vi "ER2007 Data History Panel.vi"() -> ()   [LabVIEW 2013]
uses:
  Controls/Global ER2007.vi
panel:
  in  "T = Update config":bool=TRUE
  in  "Case Constant\n(See Context Help)":bool
  in  "Match Scale":bool
  in  "Cursors 2":bool caption="Cursors"
  in  "AutoScl 2":bool=TRUE caption="AutoScale"
  in  "Cursors 1":bool caption="Cursors"
  in  "AutoScl 1":bool=TRUE caption="Auto Scale"
  in  "Log/Linear":bool
  in  "Print 2":bool
  in  "Print 1":bool
  in  "Export":bool
  out "Cell #":string="<none>"
  out "PV2 Label":string="F 2-3"
  out "Time ER2":dbl format="%.1f"
  out "ER2":dbl format="%.3f"
  out "Time ER1":dbl format="%.1f"
  out "ER1":dbl format="%.3f"
  out "Time PV2":dbl format="%.1f"
  out "Temp/Press":dbl format="%.1f"
  out "Time PV1":dbl format="%.1f"
  out "Pore Volume":dbl format="%.3f"
  out "Table":string[][](table)
  in  "Other PV's":u16(ring)=5 items=["FF 2-3", "Temp A", "Temp B", "Conf P", "Pore P", "Delta-P"]
  in  "ER 2":u16(ring)=2 items=["E-R 1-2", "E-R 1-3", "E-R 1-4", "E-R 2-3"]
  in  "ER 1":u16(ring)=3 items=["E-R 1-2", "E-R 1-3", "E-R 1-4", "E-R 2-3"]
  out "PV XY":cluster{"Y":dbl[], "Y":dbl[]}[](graph)
  in  "Exit":bool
  in  "Graph/Table":bool
  out "Resist XY":cluster{"Y":dbl[], "Y":dbl[]}[](graph)
  # "Data History"
  # "Resistivity Values"
  # "Process Values"
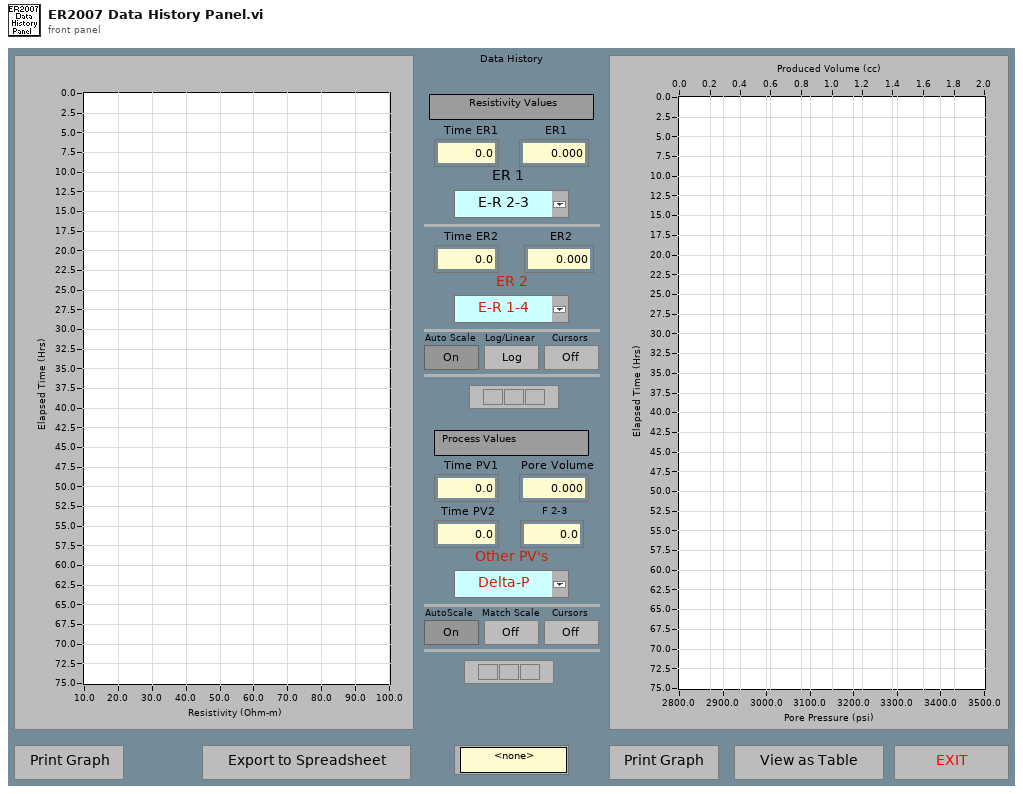
[diagram p1: front panel]
types:
  T1 = enum16{"open", "open or create", "create or replace", "create", "open (read only)"}
  T2 = cluster{"CurCell":i32, "Cell Data":cluster{"Cell ID":i32, "Cell Status":enum16{"Inactive", "Setup", "Active", "Done"}, "Project":string, "Sample #":string, "Rock Type":string, "Fluid Pair":string, "Rw":dbl, "Rw Temp":dbl, "Length":dbl, "Diameter":dbl, "Porosity":dbl, "Permeability":dbl, "4P":bool, "ElectSpace":dbl, "Frequency":dbl, "Amplitude":dbl, "DAQ Period":u32, "DAQ Units":u16, "Start Time":dbl, "Next Time":dbl, "Datafile":path, "Last Pore Vol":dbl, "Last Pore Xdcr":enum16{"<none>", "Lo Range", "Hi Range"}, "Last Resistor":enum16{"<none>", "Resistor 1", "Resistor 2", "Resistor 3", "Resistor 4", "Resistor 5", "Resistor 6"}, "CurData":dbl[][], "Comment":string}[]}
  T3 = cluster{"Cell ID":i32, "Cell Status":enum16{"Inactive", "Setup", "Active", "Done"}, "Project":string, "Sample #":string, "Rock Type":string, "Fluid Pair":string, "Rw":dbl, "Rw Temp":dbl, "Length":dbl, "Diameter":dbl, "Porosity":dbl, "Permeability":dbl, "4P":bool, "ElectSpace":dbl, "Frequency":dbl, "Amplitude":dbl, "DAQ Period":u32, "DAQ Units":u16, "Start Time":dbl, "Next Time":dbl, "Datafile":path, "Last Pore Vol":dbl, "Last Pore Xdcr":enum16{"<none>", "Lo Range", "Hi Range"}, "Last Resistor":enum16{"<none>", "Resistor 1", "Resistor 2", "Resistor 3", "Resistor 4", "Resistor 5", "Resistor 6"}, "CurData":dbl[][], "Comment":string}[]
  T4 = cluster{"Cell ID":i32, "Cell Status":enum16{"Inactive", "Setup", "Active", "Done"}, "Project":string, "Sample #":string, "Rock Type":string, "Fluid Pair":string, "Rw":dbl, "Rw Temp":dbl, "Length":dbl, "Diameter":dbl, "Porosity":dbl, "Permeability":dbl, "4P":bool, "ElectSpace":dbl, "Frequency":dbl, "Amplitude":dbl, "DAQ Period":u32, "DAQ Units":u16, "Start Time":dbl, "Next Time":dbl, "Datafile":path, "Last Pore Vol":dbl, "Last Pore Xdcr":enum16{"<none>", "Lo Range", "Hi Range"}, "Last Resistor":enum16{"<none>", "Resistor 1", "Resistor 2", "Resistor 3", "Resistor 4", "Resistor 5", "Resistor 6"}, "CurData":dbl[][], "Comment":string}
  T5 = cluster{"ER-1":u16, "ER-2":u16, "PV-Top":u16, "PV-Bot":u16, "GraphCfg":cluster{"AutoScl":bool, "T-Hi":dbl, "T-Lo":dbl, "PV-Hi":dbl, "PV-Lo":dbl}[]}
  T6 = cluster{"AutoScl":bool, "T-Hi":dbl, "T-Lo":dbl, "PV-Hi":dbl, "PV-Lo":dbl}[]
  T7 = cluster{"AutoScl":bool, "T-Hi":dbl, "T-Lo":dbl, "PV-Hi":dbl, "PV-Lo":dbl}
  T8 = typedef "LVPointDoubleTypeDef.ctl" = cluster{"Cursor X":dbl, "Cursor Y":dbl}
  T9 = typedef "LVRangeTypeDef.ctl" = cluster{"Minimum":dbl, "Maximum":dbl, "Increment":dbl, "Minor Increment":dbl, "Start":dbl}
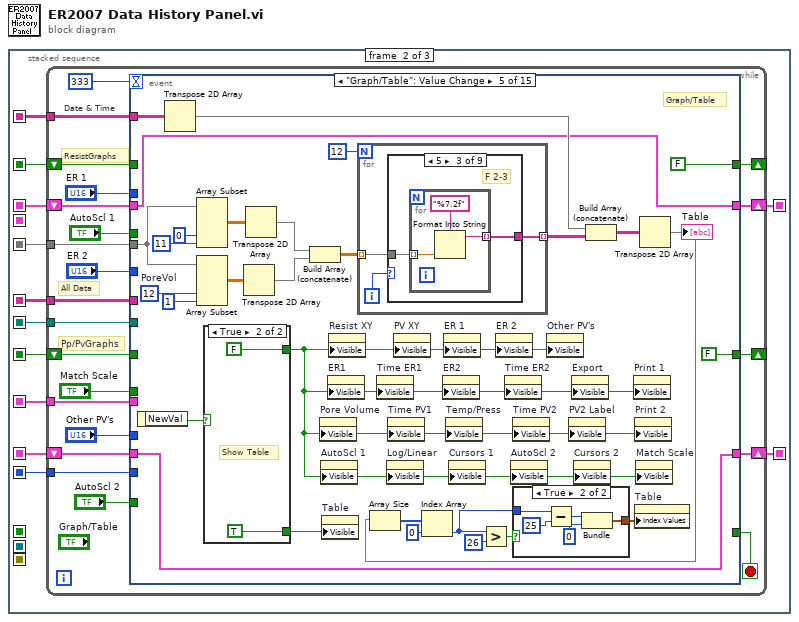
[diagram p0: block diagram]
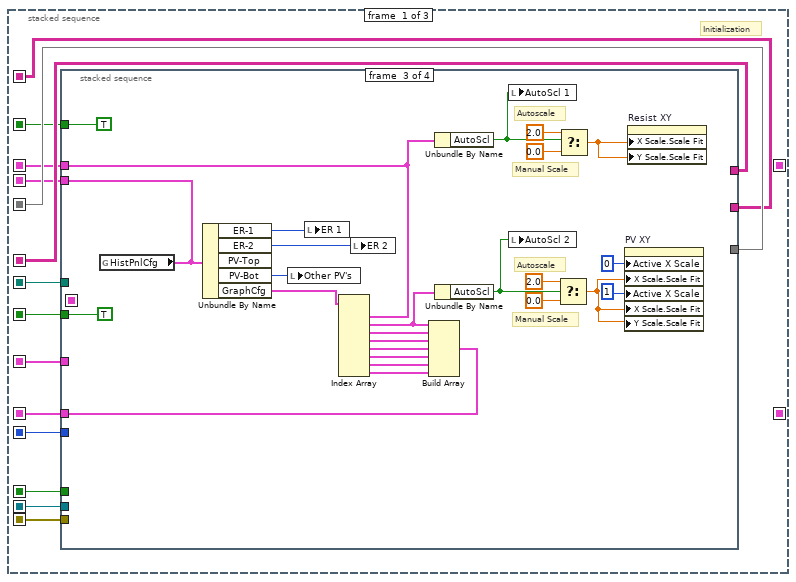
[diagram p2: hidden frame]
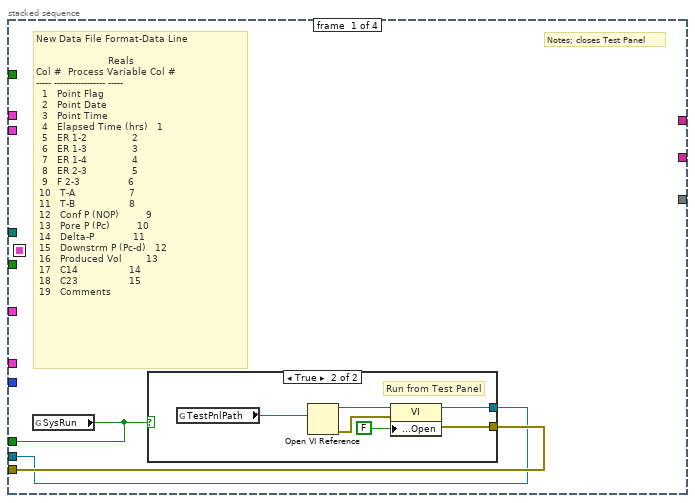
[diagram p3: hidden frame]
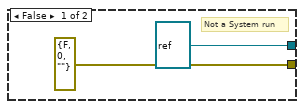
[diagram p4: hidden frame]
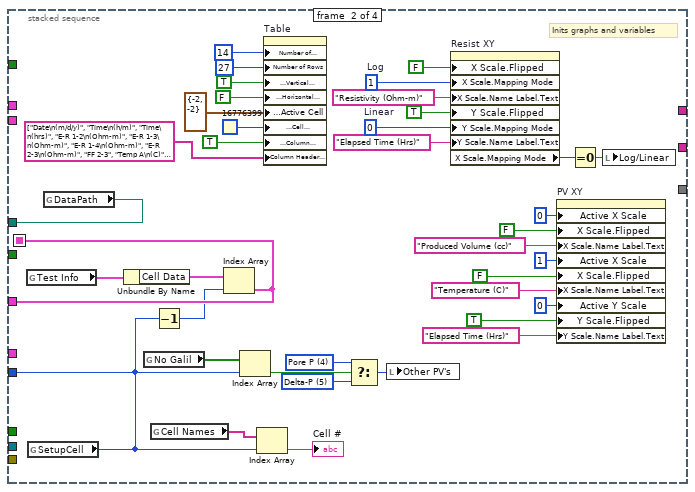
[diagram p5: hidden frame]
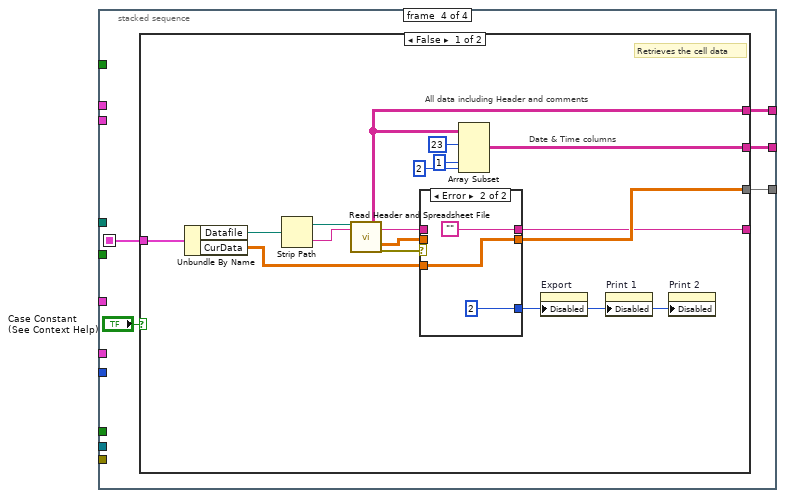
[diagram p6: hidden frame]
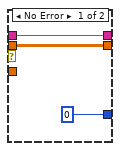
[diagram p7: hidden frame]
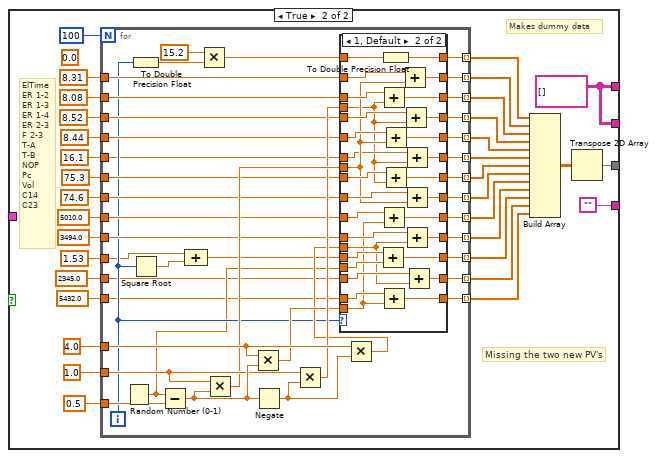
[diagram p8: hidden frame]
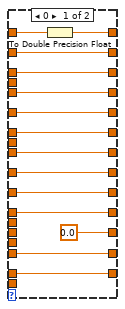
[diagram p9: hidden frame]
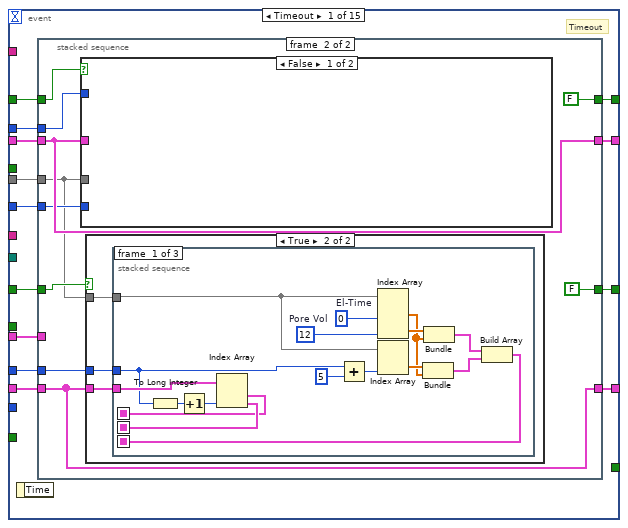
[diagram p10: hidden frame]
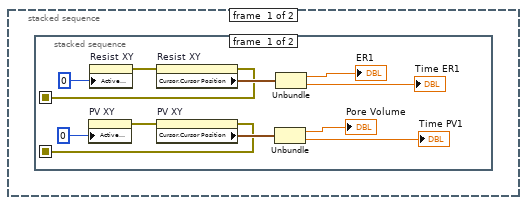
[diagram p11: hidden frame]
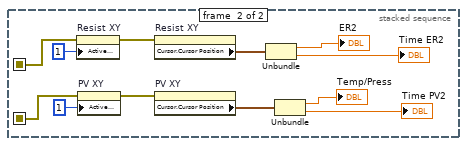
[diagram p12: hidden frame]
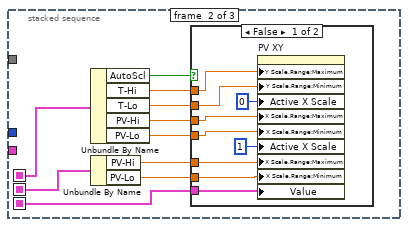
[diagram p14: hidden frame]
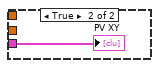
[diagram p15: hidden frame]
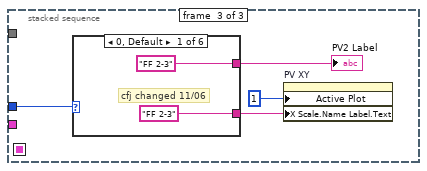
[diagram p16: hidden frame]
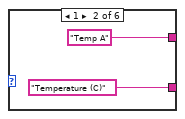
[diagram p17: hidden frame]
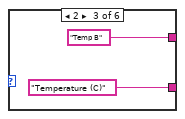
[diagram p18: hidden frame]
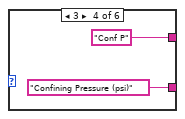
[diagram p19: hidden frame]
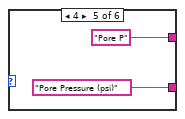
[diagram p20: hidden frame]
diagram:
  n1 = stacked-sequence {
    seq-local: [w10 _ _] -> [_ w247 _]
    seq-local: [w14 _ _] -> [_ _ w844]
    seq-local: [w13 _ _] -> [_ _ w843]
    seq-local: [w12 _ _] -> [_ _ w842]
    seq-local: [w11 _ _] -> [_ w246 _]
    seq-local: [w9 _ _] -> [_ w245 _]
    seq-local: [w8 _ _] -> [_ w244 _]
    seq-local: [w7 _ _] -> [_ w243 _]
    seq-local: [w6 _ _] -> [_ w242 _]
    seq-local: [w5 _ _] -> [_ _ w841]
    seq-local: [w2 _ _] -> [_ w240 _]
    seq-local: [w4 _ _] -> [_ w239 _]
    seq-local: [w3 _ _] -> [_ w241 _]
    seq-local: [w1 _ _] -> [_ w238 _]
    seq-local: [_ w236 _] -> [_ _ w840]
    seq-local: [_ w237 _] -> [_ _ w839]
    frame #0 {
      # "Initialization"
      n2 = stacked-sequence {
        seq-local: [_ w43 _ _] -> [_ _ _ w92]
        tunnel: [_ _ _ w94] -> w10
        tunnel: [w16 _ _ _] -> w14
        tunnel: [w15 _ _ _] -> w13
        tunnel: [w17 _ _ _] -> w12
        tunnel: [_ w43 _ _] -> w11
        tunnel: [_ w30 _ _] -> w9
        tunnel: [_ w40 _ _] -> w8
        tunnel: [_ _ _ w91] -> w7
        tunnel: [_ _ _ w90] -> w6
        tunnel: [_ _ w89 _] -> w5
        tunnel: [_ _ TRUE _] -> w4
        tunnel: [_ _ TRUE _] -> w3
        tunnel: [_ _ w82 _] -> w2
        tunnel: [_ _ w74 _] -> w1
        frame #0 {
          # "New Data File Format-Data Line\n\n                        Reals\nCol #  Process Variable Col #\n----- ----------------- -----\n  1   Point Flag\n  2   Point Date\n  3   Point Time\n  4   Elapsed Time (hrs)   1\n  5   ER 1-2               2\n  6   ER 1-3               3\n  7   ER 1-4               4\n  8   ER 2-3               5\n  9   F 2-3                6\n 10   T-A                  7\n 11   T-B                  8\n 12   Conf P (NOP)         9\n 13   Pore P (Pc)         10\n 14   Delta-P             11\n 15   Downstrm P (Pc-d)   12\n 16   Produced Vol        13\n 17   C14                 14\n 18   C23                 15\n 19   Comments"
          # "Notes; closes Test Panel"
          n3 = global read "Global ER2007.vi" "SysRun"() -> (w16:bool)
          n4 = case shown="True" w16 {
            tunnel: [refnum<vi> refnum w22] -> w15
            tunnel: [errorcluster {"status"=FALSE, "code"=0, "source"=""} ("error out") w21] -> w17
            frame False {
              # "Not a System run"
            }
            frame True {
              # "Run from Test Panel"
              n5 = global read "Global ER2007.vi" "TestPnlPath"() -> (w20:path)
              n6 = Open VI Reference(vi path=w20) -> (vi reference=w25:refnum<vi>, error out=w24:errorcluster)  [unwired: 5 in]
              n7 = property class="VI"(reference=w25, error in=w24, "Front Panel Window:Open"=FALSE) -> (reference out=w22:refnum<vi>, error out=w21:errorcluster)
            }
          }
        }
        frame #1 {
          w28 = u16 4 items=["FF 2-3", "Temp A", "Temp B", "Conf P", "Pore P", "Delta-P"] ("Other PV's")
          w27 = u16 5 items=["FF 2-3", "Temp A", "Temp B", "Conf P", "Pore P", "Delta-P"] ("Other PV's")
          w54 = u8 0  # Linear
          w55 = u8 1  # Log
          # "Inits graphs and variables"
          n8 = global read "Global ER2007.vi" "Test Info"() -> (w39:T2)
          n9 = global read "Global ER2007.vi" "SetupCell"() -> (w30:i32)
          n10 = global read "Global ER2007.vi" "DataPath"() -> (w40:path)
          n11 = Unbundle By Name(w39) -> ("Cell Data"=w44:T3)
          n12 = global read "Global ER2007.vi" "No Galil"() -> (w31:bool[])
          n13 = global read "Global ER2007.vi" "Cell Names"() -> (w38:string[])
          n14 = Decrement(x=w30) -> (x-1=w36:i32)
          n15 = Index Array(array=w44, index=w36) -> (element=w43:T4)
          n16 = Index Array(array=w31, index=w30) -> (element=w29:bool)
          n17 = Index Array(array=w38, index=w30) -> (element=→"Cell #":string)
          n18 = property on="Table" class="Tbl (strict)"("Number of Columns"=u32 14, "Number of Rows"=u32 27, "Visible Items:Vertical Scrollbar Visible"=TRUE ("Vertical Scrollbar Visible"), "Visible Items:Horizontal Scrollbar Visible"=FALSE ("Horizontal Scrollbar Visible"), "Active Cell:Active Cell"=cluster{"Row":i32, "Column":i32} {"Row"=-2, "Column"=-2} ("Active Cell"), "Active Cell:Cell Background Color"=u32 16776399, "Visible Items:Column Headers Visible"=TRUE ("Column Headers Visible"), "Column Header Strings[]"=string[] ["Date\n(m/d/y)", "Time\n(h/m)", "Time\n(hrs)", "E-R 1-2\n(Ohm-m)", "E-R 1-3\n(Ohm-m)", "E-R 1-4\n(Ohm-m)", "E-R 2-3\n(Ohm-m)", "FF 2-3", "Temp A\n(C)", "Temp B\n(C)", "Conf P\n(psi)", "Pore P\n(psi)", "Delta-P\n(psi)", "Prod Vol\n(cc)"] ("Column Headers[]")) -> ()  [unwired: 2 in, 2 out]
          n19 = Select(t=w28, s=w29, f=w27) -> (s? t:f=w26:u16)
          n20 = local write "Other PV's"(w26) -> ()
          n21 = property on="Resist XY" class="XYGraph (strict)"("X Scale.Flipped"=FALSE, "X Scale.Mapping Mode"=w55, "X Scale.Name Label.Text"="Resistivity (Ohm-m)", "Y Scale.Flipped"=TRUE, "Y Scale.Mapping Mode"=w54, "Y Scale.Name Label.Text"="Elapsed Time (Hrs)") -> ("X Scale.Mapping Mode"=w41:u8)  [unwired: 2 in, 2 out]
          n22 = property on="PV XY" class="XYGraph (strict)"("Active X Scale"=0, "X Scale.Flipped"=FALSE, "X Scale.Name Label.Text"="Produced Volume (cc)", "Active X Scale"=1, "X Scale.Flipped"=FALSE, "X Scale.Name Label.Text"="Temperature (C)", "Active Y Scale"=0, "Y Scale.Flipped"=TRUE, "Y Scale.Name Label.Text"="Elapsed Time (Hrs)") -> ()  [unwired: 2 in, 2 out]
          n23 = Equal To 0?(x=w41) -> (x = 0?=w42:bool)
          n24 = local write "Log/Linear"(w42) -> ()
        }
        frame #2 {
          # "Manual Scale"
          # "Manual Scale"
          # "Autoscale"
          # "Autoscale"
          n25 = global read "Global ER2007.vi" "HistPnlCfg"() -> (w89:T5)
          n26 = Unbundle By Name(w89) -> ("ER-1"=w86:u16, "ER-2"=w85:u16, "PV-Bot"=w84:u16, "GraphCfg"=w83:T6)  [unwired: 1 out]
          n27 = local write "Other PV's"(w84) -> ()
          n28 = local write "ER 1"(w86) -> ()
          n29 = Index Array(array=w83) -> (element #1=w82:T7, element #2=w75:T7, element #3=w81:T7, element #4=w80:T7, element #5=w79:T7, element #6=w78:T7, element #7=w77:T7, element #8=w76:T7)  [unwired: 8 in]
          n30 = local write "ER 2"(w85) -> ()
          n31 = Build Array(w75, w81, w80, w79, w78, w77, w76) -> (w74:T6)
          n32 = Unbundle By Name(w82) -> ("AutoScl"=w69:bool)
          n33 = Unbundle By Name(w75) -> ("AutoScl"=w68:bool)
          n34 = local write "AutoScl 1"(w69) -> ()
          n35 = local write "AutoScl 2"(w68) -> ()
          n36 = Select(t=2.0, s=w68, f=0.0) -> (s? t:f=w64:dbl)
          n37 = Select(t=2.0, s=w69, f=0.0) -> (s? t:f=w67:dbl)
          n38 = property on="PV XY" class="XYGraph (strict)"("Active X Scale"=0, "X Scale.Scale Fit"=w64, "Active X Scale"=1, "X Scale.Scale Fit"=w64, "Y Scale.Scale Fit"=w64) -> ()  [unwired: 2 in, 2 out]
          n39 = property on="Resist XY" class="XYGraph (strict)"("X Scale.Scale Fit"=w67, "Y Scale.Scale Fit"=w67) -> ()  [unwired: 2 in, 2 out]
        }
        frame #3 {
          n40 = case shown="False" "Case Constant\n(See Context Help)" {
            tunnel: [w102 w126] -> w94
            tunnel: w92 -> [w110 _]
            tunnel: [w101 ""] -> _
            tunnel: [w96 w117] -> w91
            tunnel: [w95 w117] -> w90
            frame False {
              # "All data including Header and comments"
              # "Date & Time columns"
              # "Retrieves the cell data"
              n41 = Unbundle By Name(w110) -> ("Datafile"=w109:path, "CurData"=w104:dbl[][])
              n42 = Strip Path(path=w109) -> (stripped path=w108:path, name=w107:string)
              n43 = call "Read Header and Spreadsheet File.vi"("DirIn"=w108, "NameIn"=w107) -> ("Table Out"=w96:string[][], "File Text Out"=w103:string, "2D Data"=w105:sgl[][], "Error Out"=w106:errorcluster)  [unwired: 11 in, 3 out]
              n44 = case shown="Error" w106 {
                tunnel: [w113 w116] -> w102
                tunnel: w105 -> [w113 _]
                tunnel: w104 -> [_ w116]
                tunnel: w103 -> [w112 _]
                tunnel: [w112 ""] -> w101
                tunnel: [u8 0 ("Disabled") u8 2 ("Disabled")] -> w100
                frame No Error {
                }
                frame Error {
                }
              }
              n45 = Array Subset(array=w96, index (row)=23 ("index"), index (col)=1 ("index"), length (col)=2 ("length")) -> (w95:string[][])  [unwired: 1 in]
              n46 = property on="Export" class="Bool"("Disabled"=w100) -> ()  [unwired: 2 in, 2 out]
              n47 = property on="Print 1" class="Bool"("Disabled"=w100) -> ()  [unwired: 2 in, 2 out]
              n48 = property on="Print 2" class="Bool"("Disabled"=w100) -> ()  [unwired: 2 in, 2 out]
            }
            frame True {
              w117 = string[][] [] ("Table Out")
              (unwired) 0.0 ("y")
              # "Missing the two new PV's"
              # "Makes dummy data"
              # "ElTime\nER 1-2\nER 1-3\nER 1-4\nER 2-3\nF 2-3\nT-A\nT-B\nNOP\nPc\nVol\nC14\nC23"
              n49 = for {
                N: 100 -> [_]
                tunnel: 0.5 ("y") -> [w190]
                tunnel: 1.0 ("y") -> [w188]
                tunnel: 4.0 ("y") -> [w187]
                tunnel: [w185] -> w131 mode=indexing
                tunnel: 8.31 ("y") -> [w181]
                tunnel: [w180] -> w130 mode=indexing
                tunnel: 8.08 ("y") -> [w178]
                tunnel: [w177] -> w129 mode=indexing
                tunnel: 8.52 ("y") -> [w175]
                tunnel: [w174] -> w128 mode=indexing
                tunnel: 8.44 ("y") -> [w173]
                tunnel: [w172] -> w137 mode=indexing
                tunnel: 75.3 ("y") -> [w171]
                tunnel: [w170] -> w136 mode=indexing
                tunnel: 74.6 ("y") -> [w169]
                tunnel: [w168] -> w135 mode=indexing
                tunnel: 5010.0 ("y") -> [w167]
                tunnel: [w166] -> w134 mode=indexing
                tunnel: 3494.0 ("y") -> [w165]
                tunnel: [w164] -> w133 mode=indexing
                tunnel: [w163] -> w132 mode=indexing
                tunnel: 1.53 ("value") -> [w156]
                tunnel: 16.1 ("y") -> [w155]
                tunnel: [w154] -> w123 mode=indexing
                tunnel: 2345.0 ("value") -> [w153]
                tunnel: 5432.0 ("value") -> [w152]
                tunnel: [w151] -> w120 mode=indexing
                tunnel: [w150] -> w119 mode=indexing
                i -> [w159]
                n50 = Random Number (0-1)() -> (number: 0 to 1=w157:dbl)
                n51 = To Double Precision Float(number=w159) -> (double precision float=w182:dbl)
                n52 = Square Root(x=w159) -> (sqrt(x)=w158:dbl)
                n53 = Subtract(x=w157, y=w190) -> (x-y=w189:dbl)
                n54 = Compound Arithmetic op=ADD(w156, w158) -> (w160:dbl)
                n55 = Multiply(x=15.2, y=w182) -> (x*y=w184:dbl)
                n56 = Multiply(x=w188, y=w189) -> (x*y=w179:dbl)
                n57 = Multiply(x=w187, y=w189) -> (x*y=w162:dbl)
                n58 = Negate(x=w189) -> (-x=w186:dbl)
                n59 = Multiply(x=w188, y=w186) -> (x*y=w176:dbl)
                n60 = Multiply(x=w187, y=w186) -> (x*y=w161:dbl)
                n61 = case shown="1, Default" w159 {
                  tunnel: w184 -> [w204 w235]
                  tunnel: [w203 w234] -> w185
                  tunnel: w181 -> [w202 w232]
                  tunnel: [w202 w233] -> w180
                  tunnel: w179 -> [_ w221]
                  tunnel: w178 -> [w201 w230]
                  tunnel: [w201 w231] -> w177
                  tunnel: w176 -> [_ w213]
                  tunnel: w175 -> [w200 w228]
                  tunnel: [w200 w229] -> w174
                  tunnel: w173 -> [w199 w226]
                  tunnel: [w199 w227] -> w172
                  tunnel: w171 -> [w198 w224]
                  tunnel: [w198 w225] -> w170
                  tunnel: w169 -> [w197 w222]
                  tunnel: [w197 w223] -> w168
                  tunnel: w167 -> [w196 w219]
                  tunnel: [w196 w220] -> w166
                  tunnel: w165 -> [w195 w217]
                  tunnel: [w195 w218] -> w164
                  tunnel: w160 -> [_ w216]
                  tunnel: [0.0 w211] -> w163
                  tunnel: w162 -> [_ w205]
                  tunnel: w161 -> [_ w206]
                  tunnel: w157 -> [_ w215]
                  tunnel: w155 -> [w191 w214]
                  tunnel: [w191 w212] -> w154
                  tunnel: w153 -> [w193 w210]
                  tunnel: w152 -> [w192 w209]
                  tunnel: [w193 w208] -> w151
                  tunnel: [w192 w207] -> w150
                  frame 0 {
                    n62 = To Double Precision Float(number=w204) -> (double precision float=w203:dbl)
                  }
                  frame 1, Default {
                    n63 = Add(x=w216, y=w215) -> (x+y=w211:dbl)
                    n64 = Add(x=w230, y=w213) -> (x+y=w231:dbl)
                    n65 = Add(x=w219, y=w205) -> (x+y=w220:dbl)
                    n66 = Add(x=w209, y=w205) -> (x+y=w207:dbl)
                    n67 = To Double Precision Float(number=w235) -> (double precision float=w234:dbl)
                    n68 = Add(x=w226, y=w221) -> (x+y=w227:dbl)
                    n69 = Add(x=w224, y=w213) -> (x+y=w225:dbl)
                    n70 = Add(x=w232, y=w221) -> (x+y=w233:dbl)
                    n71 = Add(x=w228, y=w213) -> (x+y=w229:dbl)
                    n72 = Add(x=w214, y=w213) -> (x+y=w212:dbl)
                    n73 = Add(x=w222, y=w221) -> (x+y=w223:dbl)
                    n74 = Add(x=w217, y=w206) -> (x+y=w218:dbl)
                    n75 = Add(x=w210, y=w206) -> (x+y=w208:dbl)
                  }
                }
              }
              n76 = Build Array(w131, w130, w129, w128, w137, w123, w136, w135, w134, w133, w132, w120, w119) -> (w127:dbl[][])
              n77 = Transpose 2D Array(2D array=w127) -> (transposed array=w126:dbl[][])
            }
          }
        }
      }
    }
    frame #1 {
      n78 = while {
        shift-right: [w267] -> _
        shift-left: w241 -> [w266]
        tunnel: w247 -> [w265]
        shift-right: [w262] -> _
        shift-left: w239 -> [w260]
        tunnel: w245 -> [w258]
        tunnel: w244 -> [w257]
        tunnel: w243 -> [w256]
        tunnel: w242 -> [w254]
        shift-right: [w249] -> w236
        shift-left: w240 -> [w253]
        shift-right: [w248] -> w237
        shift-left: w238 -> [w250]
        tunnel: w246 -> [w259]
        stop <- w268 stop-if-true
        # "Pp/PvGraphs"
        # "All Data"
        # "ResistGraphs"
        # "Date & Time"
        n79 = event shown="[4] \"Graph/Table\": Value Change" {
          selector: _ -> [_ _ _ _ _ _ _ _ _ _ _ _ _ _ _]
          dyn-events: _ -> [_ _ _ _ _ _ _ _ _ _ _ _ _ _ _]
          timeout: 333 -> [_ _ _ _ _ _ _ _ _ _ _ _ _ _ _]
          tunnel: [_ _ _ _ _ _ _ _ _ _ _ _ _ _ "Exit"] -> w268
          tunnel: [w273 TRUE TRUE FALSE FALSE w540 TRUE TRUE TRUE w645 w739 w750 w769 w787 FALSE] -> w267
          tunnel: w266 -> [w282 _ _ _ _ w540 _ _ _ w645 w739 w750 w769 w787 _]
          tunnel: w265 -> [w279 _ _ _ w469 _ _ _ _ _ _ _ _ _ _]
          tunnel: "ER 1" -> [w281 _ _ _ _ _ _ _ _ _ _ _ _ _ _]
          tunnel: "ER 2" -> [w278 _ _ _ _ _ _ _ _ _ _ _ _ _ _]
          tunnel: [w270 FALSE FALSE TRUE FALSE w539 w581 w604 w630 TRUE TRUE w749 w770 w788 FALSE] -> w262
          tunnel: "Other PV's" -> [w277 _ _ w425 _ _ _ _ _ w641 _ _ _ _ w792]
          tunnel: w260 -> [w272 _ _ _ _ w539 w581 w604 w630 _ _ w749 w770 w788 _]
          tunnel: w259 -> [w276 _ _ _ _ w538 _ _ _ _ _ w747 w766 _ _]
          tunnel: w258 -> [_ _ _ _ _ _ _ _ _ _ _ w748 w768 _ _]
          tunnel: w257 -> [_ _ _ _ _ _ _ _ _ _ _ w746 w767 _ _]
          tunnel: w256 -> [_ _ _ _ _ w536 _ _ _ _ _ _ _ _ _]
          tunnel: "Match Scale" -> [_ _ _ _ _ _ _ _ _ _ _ _ _ _ _]
          tunnel: w254 -> [_ _ _ _ w461 _ _ _ _ _ _ _ _ _ _]
          tunnel: w253 -> [w280 w398 w412 w427 w456 w534 w574 w598 w632 w644 w734 w745 w765 w784 w800]
          tunnel: "AutoScl 1" -> [_ w399 w413 _ _ _ _ _ _ _ _ _ _ _ _]
          tunnel: "AutoScl 2" -> [_ _ _ w426 _ _ _ _ _ _ _ _ _ _ w793]
          tunnel: w250 -> [w275 w400 w410 w424 w457 w535 w575 w599 w631 w642 w735 w744 w764 w785 w791]
          tunnel: [w274 w397 w411 w427 w456 w534 w574 w582 w632 w644 w734 w745 w765 w784 w794] -> w249
          tunnel: [w271 w400 w410 w423 w457 w535 w575 w599 w631 w640 w735 w744 w764 w785 w790] -> w248
          event Timeout {
            # "Timeout"
            n80 = event-data() -> ()  [unwired: 1 in, 1 out]
            n81 = stacked-sequence {
              tunnel: w282 -> [_ w316]
              tunnel: w281 -> [_ w315]
              tunnel: w280 -> [_ w314]
              tunnel: w279 -> [_ w309]
              tunnel: w278 -> [_ w313]
              tunnel: w277 -> [_ w310]
              tunnel: w276 -> [_ _]
              tunnel: w275 -> [_ w308]
              tunnel: [_ w314] -> w274
              tunnel: [_ FALSE] -> w273
              tunnel: w272 -> [_ w311]
              tunnel: [_ w308] -> w271
              tunnel: [_ FALSE] -> w270
              frame #0 {
                n82 = stacked-sequence {
                  seq-local: [w288 _] -> [_ w306]
                  seq-local: [w287 _] -> [_ w302]
                  frame #0 {
                    n83 = property on="PV XY" class="XYGraph (strict)"("Active Cursor"=u32 0) -> (error out=w290:errorcluster)  [unwired: 2 in, 1 out]
                    n84 = property on="Resist XY" class="XYGraph (strict)"("Active Cursor"=u32 0) -> (error out=w293:errorcluster)  [unwired: 2 in, 1 out]
                    n85 = property on="Resist XY" class="XYGraph (strict)"(error in=w293) -> (error out=w288:errorcluster, "Cursor.Cursor Position"=w292:T8)  [unwired: 1 in, 1 out]
                    n86 = property on="PV XY" class="XYGraph (strict)"(error in=w290) -> (error out=w287:errorcluster, "Cursor.Cursor Position"=w289:T8)  [unwired: 1 in, 1 out]
                    n87 = Unbundle(w289) -> ("Cursor X"=→"Pore Volume":dbl, "Cursor Y"=→"Time PV1":dbl)
                    n88 = Unbundle(w292) -> ("Cursor X"=→"ER1":dbl, "Cursor Y"=→"Time ER1":dbl)
                  }
                  frame #1 {
                    n89 = property on="Resist XY" class="XYGraph (strict)"(error in=w306, "Active Cursor"=u32 1) -> (error out=w304:errorcluster)  [unwired: 1 in, 1 out]
                    n90 = property on="PV XY" class="XYGraph (strict)"(error in=w302, "Active Cursor"=u32 1) -> (error out=w300:errorcluster)  [unwired: 1 in, 1 out]
                    n91 = property on="Resist XY" class="XYGraph (strict)"(error in=w304) -> ("Cursor.Cursor Position"=w303:T8)  [unwired: 1 in, 2 out]
                    n92 = property on="PV XY" class="XYGraph (strict)"(error in=w300) -> ("Cursor.Cursor Position"=w299:T8)  [unwired: 1 in, 2 out]
                    n93 = Unbundle(w303) -> ("Cursor X"=→"ER2":dbl, "Cursor Y"=→"Time ER2":dbl)
                    n94 = Unbundle(w299) -> ("Cursor X"=→"Temp/Press":dbl, "Cursor Y"=→"Time PV2":dbl)
                  }
                }
              }
              frame #1 {
                n95 = case shown="False" w316 {
                  tunnel: w315 -> [_ w386]
                  tunnel: w314 -> [_ w390]
                  tunnel: w309 -> [_ w383]
                  tunnel: w313 -> [_ w385]
                  frame False {
                  }
                  frame True {
                    w387 = 0  # El-Time
                    n96 = Increment(x=w385) -> (x+1=w384:u16)
                    n97 = Increment(x=w386) -> (x+1=w388:u16)
                    n98 = Index Array(array=w383, index (col)=w384) -> (element=w382:dbl[])  [unwired: 1 in]
                    n99 = Index Array(array=w383, index (col) #1=w387, index (col) #2=w388) -> (element #1=w379:dbl[], element #2=w389:dbl[])  [unwired: 2 in]
                    n100 = Bundle("CurData"=w382, "CurData"=w379) -> (w380:cluster{"CurData":dbl[], "CurData":dbl[]})  [unwired: 1 in]
                    n101 = Bundle("CurData"=w389, "CurData"=w379) -> (w381:cluster{"CurData":dbl[], "CurData":dbl[]})  [unwired: 1 in]
                    n102 = Build Array(w381, w380) -> (w373:cluster{"CurData":dbl[], "CurData":dbl[]}[])
                    n103 = Unbundle By Name(w390) -> ("AutoScl"=w378:bool, "T-Hi"=w377:dbl, "T-Lo"=w376:dbl, "PV-Hi"=w375:dbl, "PV-Lo"=w374:dbl)
                    n104 = case shown="False" w378 {
                      tunnel: w377 -> [w395 _]
                      tunnel: w376 -> [w394 _]
                      tunnel: w375 -> [w393 _]
                      tunnel: w374 -> [w392 _]
                      tunnel: w373 -> [w391 w396]
                      frame False {
                        n105 = property on="Resist XY" class="XYGraph (strict)"("Y Scale.Range:Maximum"=w395, "Y Scale.Range:Minimum"=w394, "X Scale.Range:Maximum"=w393, "X Scale.Range:Minimum"=w392, "Value"=w391) -> ()  [unwired: 2 in, 2 out]
                      }
                      frame True {
                        "Resist XY" <- w396
                      }
                    }
                  }
                }
                n106 = case shown="True" w311 {
                  tunnel: w310 -> [_ w318]
                  tunnel: w308 -> [_ w317]
                  tunnel: w309 -> [_ w319]
                  frame False {
                  }
                  frame True {
                    n107 = stacked-sequence {
                      seq-local: [w326 _ _] -> [_ w337 _]
                      seq-local: [w323 _ _] -> [_ w345 _]
                      seq-local: [w322 _ _] -> [_ w346 _]
                      tunnel: w319 -> [w327 _ _]
                      tunnel: w318 -> [w324 _ w357]
                      tunnel: w317 -> [w325 _ _]
                      frame #0 {
                        w333 = 12  # Pore Vol
                        w330 = 0  # El-Time
                        n108 = To Long Integer(number=w324) -> (32bit integer=w321:i32)
                        n109 = Increment(x=w321) -> (x+1=w320:i32)
                        n110 = Index Array(array=w325, index #2=w320) -> (element #1=w322:T7, element #2=w323:T7)  [unwired: 1 in]
                        n111 = Add(x=w324, y=u16 5) -> (x+y=w331:u16)
                        n112 = Index Array(array=w327, index (col) #1=w330, index (col) #2=w333) -> (element #1=w334:dbl[], element #2=w335:dbl[])  [unwired: 2 in]
                        n113 = Index Array(array=w327, index (col)=w331) -> (element=w336:dbl[])  [unwired: 1 in]
                        n114 = Bundle("CurData"=w336, "CurData"=w334) -> (w329:cluster{"CurData":dbl[], "CurData":dbl[]})  [unwired: 1 in]
                        n115 = Bundle("CurData"=w335, "CurData"=w334) -> (w328:cluster{"CurData":dbl[], "CurData":dbl[]})  [unwired: 1 in]
                        n116 = Build Array(w328, w329) -> (w326:cluster{"CurData":dbl[], "CurData":dbl[]}[])
                      }
                      frame #1 {
                        n117 = Unbundle By Name(w346) -> ("AutoScl"=w344:bool, "T-Hi"=w343:dbl, "T-Lo"=w342:dbl, "PV-Hi"=w341:dbl, "PV-Lo"=w340:dbl)
                        n118 = Unbundle By Name(w345) -> ("PV-Hi"=w339:dbl, "PV-Lo"=w338:dbl)
                        n119 = case shown="False" w344 {
                          tunnel: w343 -> [w355 _]
                          tunnel: w342 -> [w354 _]
                          tunnel: w341 -> [w353 _]
                          tunnel: w340 -> [w352 _]
                          tunnel: w339 -> [w349 _]
                          tunnel: w338 -> [w348 _]
                          tunnel: w337 -> [w347 w356]
                          frame False {
                            n120 = property on="PV XY" class="XYGraph (strict)"("Y Scale.Range:Maximum"=w355, "Y Scale.Range:Minimum"=w354, "Active X Scale"=0, "X Scale.Range:Maximum"=w353, "X Scale.Range:Minimum"=w352, "Active X Scale"=1, "X Scale.Range:Maximum"=w349, "X Scale.Range:Minimum"=w348, "Value"=w347) -> ()  [unwired: 2 in, 2 out]
                          }
                          frame True {
                            "PV XY" <- w356
                          }
                        }
                      }
                      frame #2 {
                        n121 = case shown="0, Default" w357 {
                          tunnel: ["FF 2-3" ("Y Scale.Name Label.Text") "Temperature (C)" ("Y Scale.Name Label.Text") "Temperature (C)" ("Y Scale.Name Label.Text") "Confining Pressure (psi)" ("Y Scale.Name Label.Text") "Pore Pressure (psi)" ("Y Scale.Name Label.Text") "Delta-P (psi)" ("Y Scale.Name Label.Text")] -> w360
                          tunnel: ["FF 2-3" ("PV2 Label") "Temp A" ("PV2 Label") "Temp B" ("PV2 Label") "Conf P" ("PV2 Label") "Pore P" ("PV2 Label") "Delta-P" ("PV2 Label")] -> w358
                          frame 0, Default {
                            # "cfj changed 11/06"
                          }
                          frame 1 {
                          }
                          frame 2 {
                          }
                          frame 3 {
                          }
                          frame 4 {
                          }
                          frame 5 {
                          }
                        }
                        "PV2 Label" <- w358
                        n122 = property on="PV XY" class="XYGraph (strict)"("Active Plot"=u32 1, "X Scale.Name Label.Text"=w360) -> ()  [unwired: 2 in, 2 out]
                      }
                    }
                  }
                }
              }
            }
          }
          event "ER 1": Value Change {
            # "ER 1"
            n123 = event-data() -> ()  [unwired: 1 in, 1 out]
            n124 = case shown="False" w399 {
              tunnel: w398 -> [w408 w409]
              tunnel: [w403 w409] -> w397
              frame False {
                n125 = property on="Resist XY" class="XYGraph (strict)"() -> ("Y Scale.Range:Maximum"=w407:dbl, "Y Scale.Range:Minimum"=w406:dbl, "X Scale.Range:Maximum"=w405:dbl, "X Scale.Range:Minimum"=w404:dbl)  [unwired: 2 in, 2 out]
                n126 = Bundle By Name(cluster=w408, "T-Hi"=w407, "T-Lo"=w406, "PV-Hi"=w405, "PV-Lo"=w404) -> (w403:T7)
              }
              frame True {
              }
            }
          }
          event "ER 2": Value Change {
            # "ER 2"
            n127 = event-data() -> ()  [unwired: 1 in, 1 out]
            n128 = case shown="True" w413 {
              tunnel: w412 -> [w421 w422]
              tunnel: [w416 w422] -> w411
              frame False {
                n129 = property on="Resist XY" class="XYGraph (strict)"() -> ("Y Scale.Range:Maximum"=w420:dbl, "Y Scale.Range:Minimum"=w419:dbl, "X Scale.Range:Maximum"=w418:dbl, "X Scale.Range:Minimum"=w417:dbl)  [unwired: 2 in, 2 out]
                n130 = Bundle By Name(cluster=w421, "T-Hi"=w420, "T-Lo"=w419, "PV-Hi"=w418, "PV-Lo"=w417) -> (w416:T7)
              }
              frame True {
              }
            }
          }
          event "Other PV's": Value Change {
            # "Temp/Press"
            n131 = event-data() -> ()  [unwired: 1 in, 1 out]
            n132 = case shown="True" w426 {
              tunnel: w425 -> [w447 _]
              tunnel: w424 -> [w435 w448]
              tunnel: [w430 w448] -> w423
              frame False {
                n133 = To Long Integer(number=w447) -> (32bit integer=w446:i32)
                n134 = Increment(x=w446) -> (x+1=w432:i32)
                n135 = Index Array(array=w435, index #2=w432) -> (element #1=w443:T7, element #2=w442:T7)  [unwired: 1 in]
                n136 = property on="PV XY" class="XYGraph (strict)"("Active X Scale"=0, "Active X Scale"=1) -> ("Y Scale.Range:Maximum"=w441:dbl, "Y Scale.Range:Minimum"=w440:dbl, "X Scale.Range:Maximum"=w439:dbl, "X Scale.Range:Minimum"=w438:dbl, "X Scale.Range:Maximum"=w437:dbl, "X Scale.Range:Minimum"=w436:dbl)  [unwired: 2 in, 2 out]
                n137 = Bundle By Name(cluster=w443, "T-Hi"=w441, "T-Lo"=w440, "PV-Hi"=w439, "PV-Lo"=w438) -> (w434:T7)
                n138 = Bundle By Name(cluster=w442, "PV-Hi"=w437, "PV-Lo"=w436) -> (w431:T7)
                n139 = Replace Array Subset(array=w435, new element #1=w434, index #1=0 ("index"), new element #2=w431, index #2=w432) -> (w430:T6)
              }
              frame True {
              }
            }
          }
          event "Graph/Table": Value Change {
            w468 = 12  # PoreVol
            # "Graph/Table"
            n140 = event-data() -> ("NewVal"=w477:bool)  [unwired: 1 in]
            n141 = Transpose 2D Array(2D array=w461) -> (transposed array=w459:string[][])
            n142 = Array Subset(array=w469, index (col)=0 ("index"), length (col)=11 ("length")) -> (w466:dbl[][])  [unwired: 2 in]
            n143 = Array Subset(array=w469, index (col)=w468, length (col)=1 ("length")) -> (w465:dbl[][])  [unwired: 2 in]
            n144 = case shown="True" w477 {
              tunnel: [TRUE ("Visible") FALSE ("Visible")] -> w472
              tunnel: [FALSE TRUE] -> w476
              frame False {
                # "Show graphs"
              }
              frame True {
                # "Show Table"
              }
            }
            n145 = Transpose 2D Array(2D array=w465) -> (transposed array=w464:dbl[][])
            n146 = Transpose 2D Array(2D array=w466) -> (transposed array=w463:dbl[][])
            n147 = Build Array (concatenate)(w463, w464) -> (w462:dbl[][])
            n148 = property on="Pore Volume" class="DigNum (strict)"("Visible"=w472) -> ()  [unwired: 2 in, 2 out]
            n149 = property on="AutoScl 1" class="Bool (strict)"("Visible"=w472) -> ()  [unwired: 2 in, 2 out]
            n150 = property on="Table" class="Tbl (strict)"("Visible"=w476) -> ()  [unwired: 2 in, 2 out]
            n151 = property on="ER1" class="DigNum (strict)"("Visible"=w472) -> ()  [unwired: 2 in, 2 out]
            n152 = property on="Resist XY" class="XYGraph (strict)"("Visible"=w472) -> ()  [unwired: 2 in, 2 out]
            n153 = for {
              N: 12 -> [_]
              tunnel: w462 -> [w485] mode=indexing
              tunnel: [w484] -> w460 mode=indexing
              i -> [w486]
              n154 = case shown="5" w486 {
                tunnel: w485 -> [w488 w493 w498 w503 w508 w513 w518 w523 w528]
                tunnel: [w487 w492 w497 w502 w507 w512 w517 w522 w527] -> w484
                frame 0 {
                  # "Time"
                  n155 = for {
                    tunnel: w488 -> [w491] mode=indexing
                    tunnel: [w489] -> w487 mode=indexing
                    n156 = Format Into String(format string="%7.2f", w491) -> (resulting string=w489:string)  [unwired: 2 in, 1 out]
                  }
                }
                frame 1..4 {
                  # "ER's"
                  n157 = for {
                    tunnel: w493 -> [w496] mode=indexing
                    tunnel: [w495] -> w492 mode=indexing
                    n158 = Format Into String(format string="%10.3f", w496) -> (resulting string=w495:string)  [unwired: 2 in, 1 out]
                  }
                }
                frame 5 {
                  # "F 2-3"
                  n159 = for {
                    tunnel: w498 -> [w501] mode=indexing
                    tunnel: [w500] -> w497 mode=indexing
                    n160 = Format Into String(format string="%7.2f", w501) -> (resulting string=w500:string)  [unwired: 2 in, 1 out]
                  }
                }
                frame 6, 7 {
                  # "Temps"
                  n161 = for {
                    tunnel: w503 -> [w506] mode=indexing
                    tunnel: [w505] -> w502 mode=indexing
                    n162 = Format Into String(format string="%6.1f", w506) -> (resulting string=w505:string)  [unwired: 2 in, 1 out]
                  }
                }
                frame 8 {
                  # "Conf P"
                  n163 = for {
                    tunnel: w508 -> [w511] mode=indexing
                    tunnel: [w510] -> w507 mode=indexing
                    n164 = Format Into String(format string="%6.0f", w511) -> (resulting string=w510:string)  [unwired: 2 in, 1 out]
                  }
                }
                frame 9 {
                  # "Pore P"
                  n165 = for {
                    tunnel: w513 -> [w516] mode=indexing
                    tunnel: [w515] -> w512 mode=indexing
                    n166 = Format Into String(format string="%6.0f", w516) -> (resulting string=w515:string)  [unwired: 2 in, 1 out]
                  }
                }
                frame 10 {
                  # "Delta-P"
                  n167 = for {
                    tunnel: w518 -> [w521] mode=indexing
                    tunnel: [w520] -> w517 mode=indexing
                    n168 = Format Into String(format string="%6.2f", w521) -> (resulting string=w520:string)  [unwired: 2 in, 1 out]
                  }
                }
                frame 11 {
                  # "Produced Vol"
                  n169 = for {
                    tunnel: w523 -> [w526] mode=indexing
                    tunnel: [w525] -> w522 mode=indexing
                    n170 = Format Into String(format string="%8.2f", w526) -> (resulting string=w525:string)  [unwired: 2 in, 1 out]
                  }
                }
                frame Default {
                  n171 = for {
                    tunnel: w528 -> [_] mode=indexing
                    tunnel: [""] -> w527 mode=indexing
                  }
                }
              }
            }
            n172 = property on="Time ER1" class="DigNum (strict)"("Visible"=w472) -> ()  [unwired: 2 in, 2 out]
            n173 = property on="Log/Linear" class="Bool (strict)"("Visible"=w472) -> ()  [unwired: 2 in, 2 out]
            n174 = property on="Time PV1" class="DigNum (strict)"("Visible"=w472) -> ()  [unwired: 2 in, 2 out]
            n175 = property on="PV XY" class="XYGraph (strict)"("Visible"=w472) -> ()  [unwired: 2 in, 2 out]
            n176 = property on="ER2" class="DigNum (strict)"("Visible"=w472) -> ()  [unwired: 2 in, 2 out]
            n177 = property on="ER 1" class="Ring (strict)"("Visible"=w472) -> ()  [unwired: 2 in, 2 out]
            n178 = property on="Temp/Press" class="DigNum (strict)"("Visible"=w472) -> ()  [unwired: 2 in, 2 out]
            n179 = property on="Cursors 1" class="Bool (strict)"("Visible"=w472) -> ()  [unwired: 2 in, 2 out]
            n180 = property on="ER 2" class="Ring (strict)"("Visible"=w472) -> ()  [unwired: 2 in, 2 out]
            n181 = property on="Time ER2" class="DigNum (strict)"("Visible"=w472) -> ()  [unwired: 2 in, 2 out]
            n182 = property on="AutoScl 2" class="Bool (strict)"("Visible"=w472) -> ()  [unwired: 2 in, 2 out]
            n183 = property on="Time PV2" class="DigNum (strict)"("Visible"=w472) -> ()  [unwired: 2 in, 2 out]
            n184 = property on="Other PV's" class="Ring (strict)"("Visible"=w472) -> ()  [unwired: 2 in, 2 out]
            n185 = property on="PV2 Label" class="Str"("Visible"=w472) -> ()  [unwired: 2 in, 2 out]
            n186 = property on="Export" class="Bool"("Visible"=w472) -> ()  [unwired: 2 in, 2 out]
            n187 = property on="Cursors 2" class="Bool (strict)"("Visible"=w472) -> ()  [unwired: 2 in, 2 out]
            n188 = Build Array (concatenate)(w459, w460) -> (w458:string[][])
            n189 = property on="Print 1" class="Bool"("Visible"=w472) -> ()  [unwired: 2 in, 2 out]
            n190 = property on="Print 2" class="Bool"("Visible"=w472) -> ()  [unwired: 2 in, 2 out]
            n191 = property on="Match Scale" class="Bool"("Visible"=w472) -> ()  [unwired: 2 in, 2 out]
            n192 = Transpose 2D Array(2D array=w458) -> (transposed array=w455:string[][])
            "Table" <- w455
            n193 = Array Size(array=w455) -> (size(s)=w451:i32[])
            n194 = Index Array(array=w451, index=0) -> (element=w450:i32)
            n195 = Greater?(x=w450, y=26) -> (0:w452:bool)
            n196 = case shown="True" w452 {
              tunnel: [cluster{i32, i32} {0, 0} w480] -> w449
              tunnel: w450 -> [_ w483]
              frame False {
              }
              frame True {
                n197 = Subtract(x=w483, y=25) -> (x-y=w481:i32)
                n198 = Bundle(w481, 0) -> (w480:cluster{i32, i32})  [unwired: 1 in]
              }
            }
            n199 = property on="Table" class="Tbl (strict)"("Index Values"=w449) -> ()  [unwired: 2 in, 2 out]
          }
          event "Export": Value Change {
            w537 = TRUE  # Got Excel ?
            # "Export"
            n200 = event-data() -> ()  [unwired: 1 in, 1 out]
            n201 = stacked-sequence {
              seq-local: [w551 _] -> [_ w565]
              seq-local: [w542 _] -> [_ w562]
              tunnel: w538 -> [_ _]
              tunnel: w537 -> [_ w564]
              tunnel: w536 -> [_ w563]
              frame #0 {
                # "TRUE = Cancelled"
                # "Opens a file dialog and traps\ncancelled messages"
                n202 = global read "Global ER2007.vi" "SS File Path"() -> (w541:path)
                n203 = call <vilib>:"Open_Create_Replace File.vi"("pattern"="*.xls", "prompt"="Specify a file", "function (open:0)"=T1."create or replace", "start path  (Not A Path)"=w541) -> ("error out"=w546:errorcluster, "new file path"=w551:path, "refnum"=w543:refnum<file>)  [unwired: 4 in, 1 out]
                n204 = Unbundle By Name(w546) -> ("status"=w547:bool, "code"=w545:i32)
                n205 = case shown="False" w547 {
                  tunnel: w545 -> [_ w561]
                  tunnel: w546 -> [w555 w558]
                  tunnel: [w555 w557] -> w544
                  tunnel: [FALSE w556] -> w542
                  frame False {
                  }
                  frame True {
                    w560 = 43  # Canceled
                    n206 = Equal?(x=w561, y=w560) -> (x = y?=w556:bool)
                    n207 = Select(t=errorcluster {"status"=FALSE, "code"=0, "source"=""} ("error out"), s=w556, f=w558) -> (s? t:f=w557:errorcluster)
                  }
                }
                n208 = case shown="False" w542 {
                  tunnel: w543 -> [w553 _]
                  tunnel: w544 -> [w552 _]
                  frame False {
                    n209 = Close File(refnum=w553, error in=w552) -> ()  [unwired: 2 out]
                  }
                  frame True {
                  }
                }
              }
              frame #1 {
                n210 = case shown="False" w562 {
                  tunnel: w565 -> [w568 _]
                  tunnel: w564 -> [w567 _]
                  tunnel: w563 -> [w566 _]
                  frame False {
                    # "No errors"
                    n211 = case shown="False" w567 {
                      tunnel: w568 -> [_ w571]
                      tunnel: w566 -> [_ w569]
                      frame False {
                        # "NO Excel"
                      }
                      frame True {
                        w572 = "Raw Data"  # Worksheet Name
                        # "Save file path"
                        # "Writes cell data to a specific\nworksheet on an Excel SS"
                        n212 = global read "Global ER2007.vi" "Excel Template Path"() -> (w570:path)
                        n213 = call "Write to Excel Worksheet.vi"("Worksheet"=w572, "File Out Path"=w571, "Table In"=w569, "Template Path"=w570) -> ("error out"=w573:errorcluster)  [unwired: 7 in]
                        n214 = call <vilib>:"Simple Error Handler.vi"("error in (no error)"=w573) -> ()  [unwired: 4 in, 5 out]
                      }
                    }
                  }
                  frame True {
                    # "Cancelled, error or\ninactive cell"
                  }
                }
              }
            }
          }
          event "Log/Linear": Value Change {
            w579 = u8 1  # Log
            w580 = u8 0  # Linear
            # "Log or Linear"
            n215 = event-data() -> ("NewVal"=w577:bool)  [unwired: 1 in]
            n216 = Select(t=w580, s=w577, f=w579) -> (s? t:f=w578:u8)
            n217 = property on="Resist XY" class="XYGraph (strict)"("X Scale.Mapping Mode"=w578) -> ()  [unwired: 2 in, 2 out]
          }
          event "AutoScl 1": Value Change {
            w603 = u8 2  # Auto Scale
            w602 = u8 0  # Manual Scale
            # "Auto scale 1"
            n218 = event-data() -> ("NewVal"=w583:bool)  [unwired: 1 in]
            n219 = Unbundle By Name(w598) -> ("T-Hi"=w595:dbl, "T-Lo"=w594:dbl, "PV-Hi"=w593:dbl, "PV-Lo"=w592:dbl)
            n220 = property on="Resist XY" class="XYGraph (strict)"() -> ("Y Scale.Range:Maximum"=w591:dbl, "Y Scale.Range:Minimum"=w590:dbl, "X Scale.Range:Maximum"=w589:dbl, "X Scale.Range:Minimum"=w588:dbl)  [unwired: 2 in, 2 out]
            n221 = Subtract(x=w595, y=w594) -> (x-y=w597:dbl)
            n222 = Less Or Equal To 0?(x=w597) -> (x <= 0?=w596:bool)
            n223 = Select(t=w603, s=w583, f=w602) -> (s? t:f=w601:u8)
            n224 = case shown="True" w596 {
              tunnel: w595 -> [w616 _]
              tunnel: w594 -> [w615 _]
              tunnel: w593 -> [w614 _]
              tunnel: w592 -> [w613 _]
              tunnel: w591 -> [w612 w629]
              tunnel: w590 -> [w611 w628]
              tunnel: w589 -> [w610 w627]
              tunnel: w588 -> [w609 w626]
              tunnel: [w608 w629] -> w587
              tunnel: [w607 w628] -> w586
              tunnel: [w606 w627] -> w585
              tunnel: [w605 w626] -> w584
              tunnel: w583 -> [w617 _]
              frame False {
                n225 = case shown="True" w617 {
                  tunnel: w616 -> [w621 _]
                  tunnel: w615 -> [w620 _]
                  tunnel: w614 -> [w619 _]
                  tunnel: w613 -> [w618 _]
                  tunnel: w612 -> [_ w625]
                  tunnel: w611 -> [_ w624]
                  tunnel: w610 -> [_ w623]
                  tunnel: w609 -> [_ w622]
                  tunnel: [w621 w625] -> w608
                  tunnel: [w620 w624] -> w607
                  tunnel: [w619 w623] -> w606
                  tunnel: [w618 w622] -> w605
                  frame False {
                    # "Going to Manual scale - \nuse previous min/max\nvalues"
                  }
                  frame True {
                    # "Going to Autoscale - \nsave current scale\nmin/max values"
                  }
                }
              }
              frame True {
                # "Not good min/max - \nget new ones"
              }
            }
            n226 = property on="Resist XY" class="XYGraph (strict)"("X Scale.Scale Fit"=w601, "Y Scale.Scale Fit"=w601) -> ()  [unwired: 2 in, 2 out]
            n227 = Bundle By Name(cluster=w598, "AutoScl"=w583, "T-Hi"=w587, "T-Lo"=w586, "PV-Hi"=w585, "PV-Lo"=w584) -> (w582:T7)
          }
          event "Cursors 1": Value Change {
            # "This wire went to a seperate output tunnel\nDeleted tunnel and wired to pp/pv - SD"
            # "Cursor 1 Off/On"
            n228 = event-data() -> ("NewVal"=w635:bool)  [unwired: 1 in]
            n229 = flat-sequence {
              tunnel: w635 -> [w637]
              tunnel: [w637] -> w634
              tunnel: w634 -> [w639]
              frame #0 {
                n230 = property on="Resist XY" class="XYGraph (strict)"("Active Cursor"=0 ("Cursor.Cursor Index"), "Cursor.Visible"=w637) -> ()  [unwired: 2 in, 2 out]
              }
              frame #1 {
                n231 = property on="Resist XY" class="XYGraph (strict)"("Active Cursor"=1 ("Cursor.Cursor Index"), "Cursor.Visible"=w639) -> ()  [unwired: 2 in, 2 out]
              }
            }
          }
          event "AutoScl 2": Value Change {
            # "Auto scale 2"
            n232 = event-data() -> ("NewVal"=w643:bool)  [unwired: 1 in]
            n233 = stacked-sequence {
              seq-local: [_ w678 _] -> [_ _ w723]
              seq-local: [_ w675 _] -> [_ _ w732]
              seq-local: [_ w676 _] -> [_ _ w733]
              seq-local: [_ w658 _] -> [_ _ w727]
              seq-local: [_ w657 _] -> [_ _ w726]
              seq-local: [_ w656 _] -> [_ _ w725]
              seq-local: [_ w655 _] -> [_ _ w724]
              seq-local: [_ w654 _] -> [_ _ w729]
              seq-local: [_ w653 _] -> [_ _ w728]
              tunnel: w643 -> [w647 w672 w730]
              tunnel: w642 -> [_ w679 w731]
              tunnel: w641 -> [_ w681 _]
              tunnel: [_ _ w719] -> w640
              frame #0 {
                w652 = u8 2  # Auto Scale
                w651 = u8 0  # Manual Scale
                n234 = Select(t=w652, s=w647, f=w651) -> (s? t:f=w648:u8)
                n235 = property on="PV XY" class="XYGraph (strict)"("Active X Scale"=0, "X Scale.Scale Fit"=w648, "Active X Scale"=1, "X Scale.Scale Fit"=w648, "Y Scale.Scale Fit"=w648) -> ()  [unwired: 2 in, 2 out]
              }
              frame #1 {
                n236 = To Long Integer(number=w681) -> (32bit integer=w680:i32)
                n237 = Increment(x=w680) -> (x+1=w678:i32)
                n238 = Index Array(array=w679, index #2=w678) -> (element #1=w676:T7, element #2=w675:T7)  [unwired: 1 in]
                n239 = Unbundle By Name(w676) -> ("T-Hi"=w664:dbl, "T-Lo"=w663:dbl, "PV-Hi"=w662:dbl, "PV-Lo"=w661:dbl)
                n240 = Unbundle By Name(w675) -> ("PV-Hi"=w660:dbl, "PV-Lo"=w659:dbl)
                n241 = property on="PV XY" class="XYGraph (strict)"("Active X Scale"=0, "Active X Scale"=1) -> ("Y Scale.Range:Maximum"=w670:dbl, "Y Scale.Range:Minimum"=w669:dbl, "X Scale.Range:Maximum"=w668:dbl, "X Scale.Range:Minimum"=w667:dbl, "X Scale.Range:Maximum"=w666:dbl, "X Scale.Range:Minimum"=w665:dbl)  [unwired: 2 in, 2 out]
                n242 = Subtract(x=w664, y=w663) -> (x-y=w674:dbl)
                n243 = Less Or Equal To 0?(x=w674) -> (x <= 0?=w673:bool)
                n244 = case shown="False" w673 {
                  tunnel: w672 -> [w700 _]
                  tunnel: w670 -> [w687 w718]
                  tunnel: w669 -> [w686 w717]
                  tunnel: w668 -> [w685 w716]
                  tunnel: w667 -> [w684 w715]
                  tunnel: w666 -> [w683 w714]
                  tunnel: w665 -> [w682 w713]
                  tunnel: w664 -> [w699 _]
                  tunnel: w663 -> [w698 _]
                  tunnel: w662 -> [w697 _]
                  tunnel: w661 -> [w696 _]
                  tunnel: w660 -> [w695 _]
                  tunnel: w659 -> [w694 _]
                  tunnel: [w693 w718] -> w658
                  tunnel: [w692 w717] -> w657
                  tunnel: [w691 w716] -> w656
                  tunnel: [w690 w715] -> w655
                  tunnel: [w689 w714] -> w654
                  tunnel: [w688 w713] -> w653
                  frame False {
                    n245 = case shown="False" w700 {
                      tunnel: w699 -> [w706 _]
                      tunnel: w698 -> [w705 _]
                      tunnel: w697 -> [w704 _]
                      tunnel: w696 -> [w703 _]
                      tunnel: w695 -> [w702 _]
                      tunnel: w694 -> [w701 _]
                      tunnel: [w706 w707] -> w693
                      tunnel: [w705 w708] -> w692
                      tunnel: [w704 w709] -> w691
                      tunnel: [w703 w710] -> w690
                      tunnel: [w702 w711] -> w689
                      tunnel: [w701 w712] -> w688
                      tunnel: w687 -> [_ w707]
                      tunnel: w686 -> [_ w708]
                      tunnel: w685 -> [_ w709]
                      tunnel: w684 -> [_ w710]
                      tunnel: w683 -> [_ w711]
                      tunnel: w682 -> [_ w712]
                      frame False {
                        # "Going from Manual scale - \nuse previous min/max\nvalues"
                      }
                      frame True {
                        # "Going to \nAutoscale - \nsave current\nmin/max \nvalues."
                      }
                    }
                  }
                  frame True {
                    # "Not good min/max values - \nget new ones"
                  }
                }
              }
              frame #2 {
                # "Reassembles the array of clusters"
                n246 = Bundle By Name(cluster=w732, "PV-Hi"=w729, "PV-Lo"=w728) -> (w722:T7)
                n247 = Bundle By Name(cluster=w733, "AutoScl"=w730, "T-Hi"=w727, "T-Lo"=w726, "PV-Hi"=w725, "PV-Lo"=w724) -> (w720:T7)
                n248 = Replace Array Subset(array=w731, new element #1=w720, index #1=0 ("index"), new element #2=w722, index #2=w723) -> (w719:T6)
              }
            }
          }
          event "Cursors 2": Value Change {
            # "Arrarys wired though - SD"
            # "Cursor 2 Off/On"
            n249 = event-data() -> ("NewVal"=w738:bool)  [unwired: 1 in]
            n250 = flat-sequence {
              tunnel: w738 -> [w740]
              tunnel: [w740] -> w737
              tunnel: w737 -> [w742]
              frame #0 {
                n251 = property on="PV XY" class="XYGraph (strict)"("Active Cursor"=u32 0, "Cursor.Visible"=w740) -> ()  [unwired: 2 in, 2 out]
              }
              frame #1 {
                n252 = property on="PV XY" class="XYGraph (strict)"("Active Cursor"=u32 1, "Cursor.Visible"=w742) -> ()  [unwired: 2 in, 2 out]
              }
            }
          }
          event "Print 1": Value Change {
            # "Arrarys wired though - SD"
            # "Print 1"
            n253 = event-data() -> ()  [unwired: 1 in, 1 out]
            n254 = stacked-sequence {
              tunnel: w748 -> [_ w755 _]
              tunnel: w747 -> [_ w760 _]
              tunnel: w746 -> [_ w759 _]
              frame #0 {
                w752 = u8 2 ("Disabled")
                n255 = property on="Resist XY" class="XYGraph (strict)"("Palette:Visible"=FALSE) -> ()  [unwired: 2 in, 2 out]
                n256 = property on="Print 1" class="Bool"("Disabled"=w752) -> ()  [unwired: 2 in, 2 out]
                n257 = property on="Print 2" class="Bool"("Disabled"=w752) -> ()  [unwired: 2 in, 2 out]
              }
              frame #1 {
                n258 = global read "Global ER2007.vi" "Cell Names"() -> (w754:string[])
                n259 = control-ref of="Resist XY"() -> (w761:refnum<vi>)
                n260 = Unbundle By Name(w760) -> ("Project"=w758:string, "Sample #"=w757:string)
                n261 = Index Array(array=w754, index=w755) -> (element=w753:string)
                n262 = call "Print Graph Image.vi"("Cell ID"=w753, "Graph Reference"=w761, "Sample"=w757, "Project"=w758, "DataPath"=w759) -> ("error out"=w756:errorcluster)  [unwired: 6 in]
                n263 = call <vilib>:"Simple Error Handler.vi"("error in (no error)"=w756) -> ()  [unwired: 4 in, 5 out]
              }
              frame #2 {
                w763 = u8 0 ("Disabled")
                n264 = property on="Print 1" class="Bool"("Disabled"=w763) -> ()  [unwired: 2 in, 2 out]
                n265 = property on="Resist XY" class="XYGraph (strict)"("Palette:Visible"=TRUE) -> ()  [unwired: 2 in, 2 out]
                n266 = property on="Print 2" class="Bool"("Disabled"=w763) -> ()  [unwired: 2 in, 2 out]
              }
            }
          }
          event "Print 2": Value Change {
            # "Arrarys wired though - SD"
            # "Print 2"
            n267 = event-data() -> ()  [unwired: 1 in, 1 out]
            n268 = stacked-sequence {
              tunnel: w768 -> [_ w774 _]
              tunnel: w767 -> [_ w778 _]
              tunnel: w766 -> [_ w777 _]
              frame #0 {
                w772 = u8 2 ("Disabled")
                n269 = property on="Print 1" class="Bool"("Disabled"=w772) -> ()  [unwired: 2 in, 2 out]
                n270 = property on="PV XY" class="XYGraph (strict)"("Palette:Visible"=FALSE) -> ()  [unwired: 2 in, 2 out]
                n271 = property on="Print 2" class="Bool"("Disabled"=w772) -> ()  [unwired: 2 in, 2 out]
              }
              frame #1 {
                n272 = global read "Global ER2007.vi" "Cell Names"() -> (w775:string[])
                n273 = control-ref of="PV XY"() -> (w776:refnum<vi>)
                n274 = Unbundle By Name(w777) -> ("Project"=w781:string, "Sample #"=w780:string)
                n275 = Index Array(array=w775, index=w774) -> (element=w773:string)
                n276 = call "Print Graph Image.vi"("Cell ID"=w773, "Graph Reference"=w776, "Sample"=w780, "Project"=w781, "DataPath"=w778) -> ("error out"=w779:errorcluster)  [unwired: 6 in]
                n277 = call <vilib>:"Simple Error Handler.vi"("error in (no error)"=w779) -> ()  [unwired: 4 in, 5 out]
              }
              frame #2 {
                w783 = u8 0 ("Disabled")
                n278 = property on="PV XY" class="XYGraph (strict)"("Palette:Visible"=TRUE) -> ()  [unwired: 2 in, 2 out]
                n279 = property on="Print 1" class="Bool"("Disabled"=w783) -> ()  [unwired: 2 in, 2 out]
                n280 = property on="Print 2" class="Bool"("Disabled"=w783) -> ()  [unwired: 2 in, 2 out]
              }
            }
          }
          event "Match Scale": Value Change {
            # "Arrarys wired though - SD"
            n281 = event-data() -> ("NewVal"=w786:bool)  [unwired: 1 in]
            n282 = case shown="False" w786 {
              frame False {
              }
              frame True {
                n283 = property on="Resist XY" class="XYGraph (strict)"() -> ("Y Scale.Range"=w789:T9)  [unwired: 2 in, 2 out]
                n284 = property on="PV XY" class="XYGraph (strict)"("Y Scale.Range"=w789) -> ()  [unwired: 2 in, 2 out]
              }
            }
          }
          event "Exit": Value Change {
            # "Exit"
            n285 = event-data() -> ()  [unwired: 1 in, 1 out]
            n286 = Unbundle By Name(w800) -> ("AutoScl"=w805:bool, "T-Hi"=w804:dbl, "T-Lo"=w803:dbl, "PV-Hi"=w802:dbl, "PV-Lo"=w801:dbl)
            n287 = case shown="False" w793 {
              tunnel: w792 -> [w827 _]
              tunnel: w791 -> [w813 w828]
              tunnel: [w809 w828] -> w790
              frame False {
                # "Autoscale is FALSE - save current scale values"
                n288 = To Long Integer(number=w827) -> (32bit integer=w826:i32)
                n289 = Increment(x=w826) -> (x+1=w812:i32)
                n290 = Index Array(array=w813, index #2=w812) -> (element #1=w823:T7, element #2=w822:T7)  [unwired: 1 in]
                n291 = property on="PV XY" class="XYGraph (strict)"("Active X Scale"=0, "Active X Scale"=1) -> ("Y Scale.Range:Maximum"=w818:dbl, "Y Scale.Range:Minimum"=w817:dbl, "X Scale.Range:Maximum"=w816:dbl, "X Scale.Range:Minimum"=w815:dbl, "X Scale.Range:Maximum"=w820:dbl, "X Scale.Range:Minimum"=w819:dbl)  [unwired: 2 in, 2 out]
                n292 = Bundle By Name(cluster=w823, "AutoScl"=FALSE, "T-Hi"=w818, "T-Lo"=w817, "PV-Hi"=w816, "PV-Lo"=w815) -> (w810:T7)
                n293 = Bundle By Name(cluster=w822, "T-Hi"=w820, "T-Lo"=w819, "AutoScl"=FALSE) -> (w811:T7)
                n294 = Replace Array Subset(array=w813, new element #1=w810, new element #2=w811, index #2=w812) -> (w809:T6)  [unwired: 1 in]
              }
              frame True {
                # "Autoscale is TRUE - use \nthe previous scale values"
              }
            }
            n295 = case shown="True" w805 {
              selector: w805 -> [w829 w838]
              tunnel: w804 -> [_ w837]
              tunnel: w803 -> [_ w836]
              tunnel: w802 -> [_ w835]
              tunnel: w801 -> [_ w834]
              tunnel: [w829 w838] -> w799
              tunnel: [w833 w837] -> w798
              tunnel: [w832 w836] -> w797
              tunnel: [w831 w835] -> w796
              tunnel: [w830 w834] -> w795
              frame False {
                n296 = property on="Resist XY" class="XYGraph (strict)"() -> ("Y Scale.Range:Maximum"=w833:dbl, "Y Scale.Range:Minimum"=w832:dbl, "X Scale.Range:Maximum"=w831:dbl, "X Scale.Range:Minimum"=w830:dbl)  [unwired: 2 in, 2 out]
              }
              frame True {
              }
            }
            n297 = Bundle By Name(cluster=w800, "AutoScl"=w799, "T-Hi"=w798, "T-Lo"=w797, "PV-Hi"=w796, "PV-Lo"=w795) -> (w794:T7)
          }
        }
      }
    }
    frame #2 {
      # "Cleanup and shutdown"
      n298 = stacked-sequence {
        tunnel: w844 -> [_ w861 w870]
        tunnel: w843 -> [_ w863 _]
        tunnel: w842 -> [_ w862 _]
        tunnel: w841 -> [w854 _ _]
        tunnel: w840 -> [w853 _ _]
        tunnel: w839 -> [w852 _ _]
        frame #0 {
          # "Updates the history panel config"
          n299 = Unbundle By Name(w854) -> ("GraphCfg"=w857:T6)
          n300 = local read "ER 2"() -> (w849:u16)
          n301 = Replace Array Subset(array=w857, new element #1=w853, index #1=0 ("index"), new element #2=w852, index #2=1 ("index")) -> (w851:T6)
          n302 = local read "Other PV's"() -> (w848:u16)
          n303 = local read "ER 1"() -> (w850:u16)
          n304 = local write "Graph/Table"(FALSE ("Graph/Table")) -> ()
          n305 = Bundle By Name(cluster=w854, "ER-1"=w850, "ER-2"=w849, "PV-Top"=u16 0, "PV-Bot"=w848, "GraphCfg"=w851) -> (w845:T5)
          n306 = case shown="True" "T = Update config" {
            tunnel: w845 -> [_ w859]
            frame False {
            }
            frame True {
              n307 = global write "Global ER2007.vi" "HistPnlCfg"(w859) -> ()
            }
          }
        }
        frame #1 {
          w860 = u8 0 ("Disabled")
          # "Opens front panel of calling vi before returning"
          n308 = case shown="True" w861 {
            tunnel: w863 -> [_ w865]
            tunnel: w862 -> [_ w864]
            frame False {
              # "Not a System run"
            }
            frame True {
              n309 = property class="VI"(reference=w865, error in=w864, "Front Panel Window:Open"=TRUE) -> (reference out=w868:refnum<vi>, error out=w867:errorcluster)
              n310 = Close Reference(reference=w868, error in (no error)=w867) -> (error out=w866:errorcluster)
              n311 = call <vilib>:"Simple Error Handler.vi"("error in (no error)"=w866) -> ()  [unwired: 4 in, 5 out]
            }
          }
          n312 = property on="Export" class="Bool"("Disabled"=w860) -> ()  [unwired: 2 in, 2 out]
          n313 = property on="Print 1" class="Bool"("Disabled"=w860) -> ()  [unwired: 2 in, 2 out]
          n314 = property on="Print 2" class="Bool"("Disabled"=w860) -> ()  [unwired: 2 in, 2 out]
        }
        frame #2 {
          n315 = case shown="True" w870 {
            frame False {
            }
            frame True {
              # "Close this panel's front panel"
              n316 = Current VI's Path() -> (path=w877:path)
              n317 = Open VI Reference(vi path=w877) -> (vi reference=w876:refnum<vi>, error out=w875:errorcluster)  [unwired: 5 in]
              n318 = property class="VI"(reference=w876, error in=w875, "Front Panel Window:Open"=FALSE) -> (reference out=w873:refnum<vi>, error out=w872:errorcluster)
              n319 = Close Reference(reference=w873, error in (no error)=w872) -> (error out=w871:errorcluster)
              n320 = call <vilib>:"Simple Error Handler.vi"("error in (no error)"=w871) -> ()  [unwired: 4 in, 5 out]
            }
          }
        }
      }
    }
  }
